vi "Communication_Handler.vi"() -> ()   [LabVIEW 2016]
panel:
  in  "Boolean 2":bool
  in  "String":string
  in  "Boolean":bool=TRUE
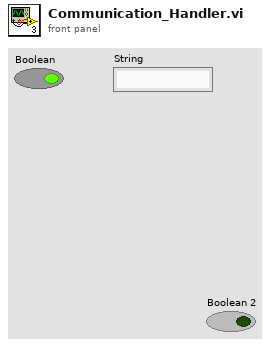
[diagram p1: front panel]
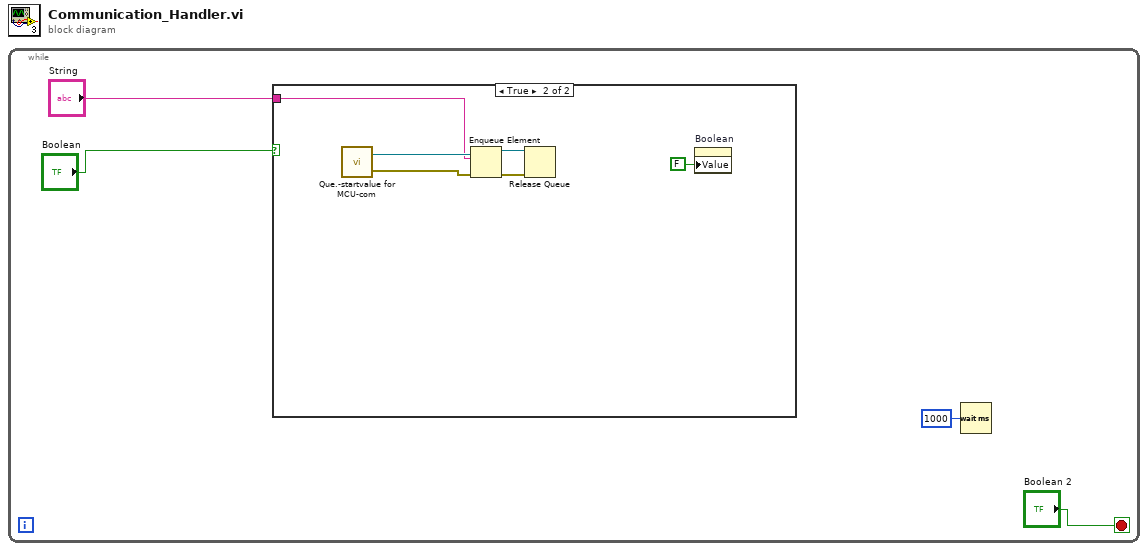
[diagram p0: block diagram]
diagram:
  n1 = while {
    stop <- "Boolean 2" stop-if-true
    n2 = case shown="True" "Boolean" {
      tunnel: "String" -> [_ w7]
      frame False {
      }
      frame True {
        n3 = call "Que.-startvalue for MCU-com.vi"() -> ("error out"=w10:errorcluster, "queue out"=w9:refnum<queue>)  [unwired: 2 in]
        n4 = Enqueue Element(queue=w9, element=w7, error in (no error)=w10) -> (queue out=w6:refnum<queue>, error out=w5:errorcluster)  [unwired: 1 in, 1 out]
        n5 = Release Queue(queue=w6, error in (no error)=w5) -> ()  [unwired: 1 in, 3 out]
        n6 = property on="Boolean" class="Bool (strict)"("Value"=FALSE ("Boolean")) -> ()  [unwired: 2 in, 2 out]
      }
    }
    n7 = Wait (ms)(milliseconds to wait=u32 1000) -> ()  [unwired: 1 out]
  }
